vi "CreatePublicEvents.vi"(8 "error in (no error)":errorcluster, 11 "RemoteControl":refnum<class "RemoteControl.lvclass">) -> (0 "error out":errorcluster, 3 "RemoteControl out":refnum<class "RemoteControl.lvclass">)   [LabVIEW 2016, in "RemoteControl.lvclass"]
doc: "---------------------------------------------------------------\nJKI State Machine Objects™\nhttp://jki.net/state-machine-objects/\nCopyright (C) 2005-2015, JKI <info@jki.net>\nALL RIGHTS RESERVEDJKI State Machine Objects (SMO) 1.0.0.4\nJKI - JKI\nCopyright (c) 2015, JKI"
uses:
  RemoteControl.lvclass
  Typedefs/PublicEvents--RemoteControl.configRemote.ctl
  Typedefs/PublicEvents--RemoteControl.configIVmode.ctl
  Typedefs/PublicEvents--RemoteControl.configREF.ctl
  Typedefs/REF-cluster.ctl
  Typedefs/REF_f-array.ctl
  Typedefs/REF_phi-array.ctl
  Typedefs/PublicEvents--RemoteControl.configAO.ctl
  Typedefs/AO-cluster.ctl
  Typedefs/AO_Amp-array.ctl
  Typedefs/AO_DC-array.ctl
  Typedefs/AO_f-array.ctl
  Typedefs/AO_phi-array.ctl
  Typedefs/Function-array.ctl
  Typedefs/Function-enum.ctl
  RemoteControl.lvclass/RemoteControl.ctl
  <vilib>/JKI/JKI SMO/SMO/SMO.lvclass
panel:
  # "For instructions on how to use the JKI State Machine Objects, examples and video tutorials, visit:\nhttp://jki.net/state-machine-objects/\n\nJKI State Machine Objects™\nhttp://jki.net/state-machine-objects/\nCopyright (C) 2005-2015, JKI <info@jki.net>\nALL RIGHTS RESERVED"
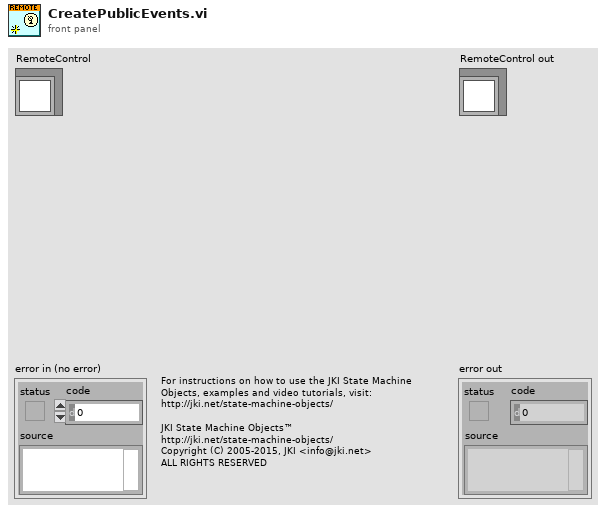
[diagram p1: front panel]
types:
  T1 = typedef "RemoteControl.lvclass/PublicEvents--RemoteControl.configAO.ctl" = cluster{"Channels: AO":T2}
  T2 = typedef "AO-cluster.ctl" = cluster{"AO amp (V)":T3, "AO DC (V)":T4, "AO f (Hz)":T5, "AO phi (deg)":T6, "function":T7}
  T3 = typedef "AO_Amp-array.ctl" = dbl[]
  T4 = typedef "AO_DC-array.ctl" = dbl[]
  T5 = typedef "AO_f-array.ctl" = dbl[]
  T6 = typedef "AO_phi-array.ctl" = dbl[]
  T7 = typedef "Function-array.ctl" = T8[]
  T8 = typedef "Function-enum.ctl" = enum16{"Sine Wave", "Triangle Wave", "Square Wave", "Sawtooth Wave"}
  T9 = typedef "RemoteControl.lvclass/PublicEvents--RemoteControl.configREF.ctl" = cluster{"Channels: Lockin":T10}
  T10 = typedef "REF-cluster.ctl" = cluster{"REF f (Hz)":T11, "REF phi (deg)":T12}
  T11 = typedef "REF_f-array.ctl" = dbl[]
  T12 = typedef "REF_phi-array.ctl" = dbl[]
  T13 = typedef "RemoteControl.lvclass/PublicEvents--RemoteControl.configIVmode.ctl" = bool
  T14 = typedef "RemoteControl.lvclass/PublicEvents--RemoteControl.configRemote.ctl" = bool
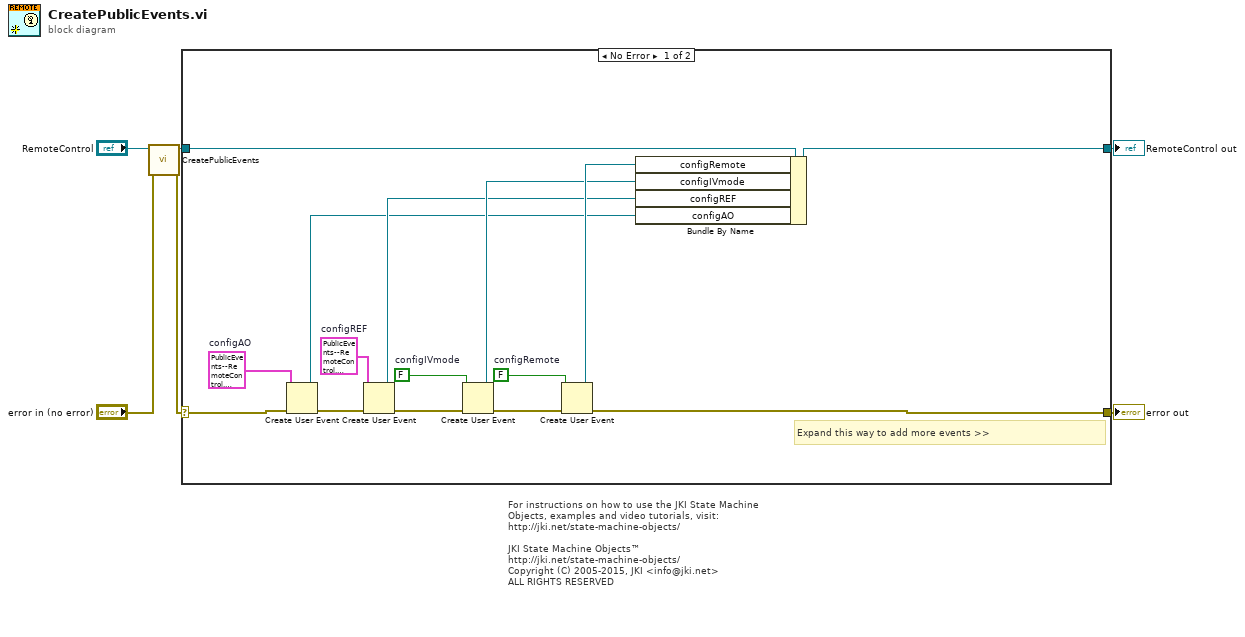
[diagram p0: block diagram]
diagram:
  # "For instructions on how to use the JKI State Machine Objects, examples and video tutorials, visit:\nhttp://jki.net/state-machine-objects/\n\nJKI State Machine Objects™\nhttp://jki.net/state-machine-objects/\nCopyright (C) 2005-2015, JKI <info@jki.net>\nALL RIGHTS RESERVED"
  n1 = call-parent "CreatePublicEvents.vi"("error in (no error)"="error in (no error)", "SMO"="RemoteControl") -> ("error out"=w1:errorcluster, "SMO out"=w3:refnum<class "RemoteControl.lvclass">)  [unwired: 8 in]
  n2 = case shown="No Error" w1 {
    selector: w1 -> [w20 w23]
    tunnel: [w18 w23] -> w5
    tunnel: [w19 w22] -> w6
    tunnel: w3 -> [w21 w22]
    frame No Error {
      w8 = T1 {"Channels: AO"={"AO amp (V)"=[0.01, 0.0, 0.0, 0.0, 0.0, 0.0, 0.0, 0.0], "AO DC (V)"=[0.0, 0.0, 0.0, 0.0, 0.0, 0.0, 0.0, 0.0], "AO f (Hz)"=[13.1, 13.0, 13.0, 13.0, 13.0, 13.0, 13.0, 13.0], "AO phi (deg)"=[0.0, 0.0, 0.0, 0.0, 0.0, 0.0, 0.0, 0.0], "function"=[enum."Sine Wave", enum."Sine Wave", enum."Sine Wave", enum."Sine Wave", enum."Sine Wave", enum."Sine Wave", enum."Sine Wave", enum."Sine Wave"]}}  # configAO
      w11 = T9 {"Channels: Lockin"={"REF f (Hz)"=[13.0], "REF phi (deg)"=[0.0, 0.0, 0.0, 0.0, 0.0, 0.0, 0.0, 0.0]}}  # configREF
      w14 = T13 FALSE  # configIVmode
      w17 = T14 FALSE  # configRemote
      # "Expand this way to add more events >>"
      n3 = Create User Event(user event datatype=w8, error in=w20) -> (user event=w7:refnum<user-event>, error out=w9:errorcluster)
      n4 = Create User Event(user event datatype=w11, error in=w9) -> (user event=w10:refnum<user-event>, error out=w12:errorcluster)
      n5 = Create User Event(user event datatype=w14, error in=w12) -> (user event=w13:refnum<user-event>, error out=w15:errorcluster)
      n6 = Create User Event(user event datatype=w17, error in=w15) -> (user event=w16:refnum<user-event>, error out=w18:errorcluster)
      n7 = Bundle By Name(cluster=w21, "configRemote"=w16, "configIVmode"=w13, "configREF"=w10, "configAO"=w7) -> (w19:refnum<class "RemoteControl.lvclass">)
    }
    frame Error {
    }
  }
  "error out" <- w5
  "RemoteControl out" <- w6
